vi "Main On Compile Action VI.vi"(8 "error in (no error)":errorcluster, 11 "Device Item Ref in":T1 format="%.0x") -> (0 "error out":errorcluster)   [LabVIEW 2014, in "SLSC configuration System Explorer.lvlib"]
uses:
  SLSC configuration System Explorer.lvlib
  <vilib>/NI Veristand/Custom Device API/Custom Device Item Ref.ctl
  Shared/Type Defs/SLSC compiled.ctl
  Shared/Type Defs/Res Sim compiled.ctl
  Shared/Type Defs/RT Engine Data.ctl
  Shared/Type Defs/RT IDs.ctl
  Shared/SPI Utility/Slot #.ctl
  Shared/MCP23S17/Chip Address.ctl
  Shared/Constants.vi
  <vilib>/NI Veristand/Custom Device API/Set Item Property (Variant).vi
  <vilib>/NI Veristand/Custom Device API/Custom Device API.lvlib
  Shared/SLSC configuration Shared.lvlib
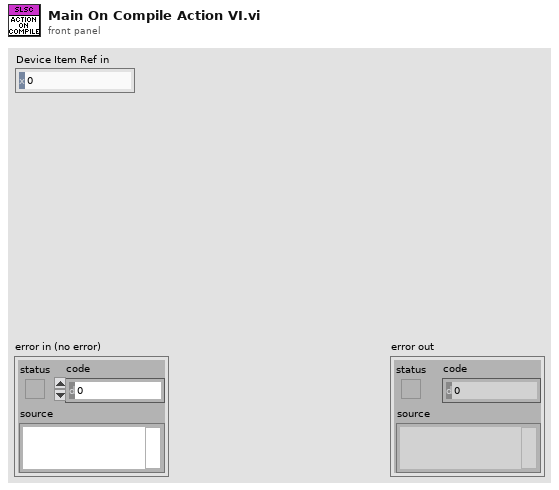
[diagram p1: front panel]
types:
  T1 = typedef "Custom Device API.lvlib/Custom Device Item Ref.ctl" = u64
  T2 = typedef "SLSC configuration Shared.lvlib/SLSC compiled.ctl" = cluster{"Initial SPI CMDs":u64[], "Res Sim data ":T3[], "Res Sim init FIFO elements":u32[], "FIU Engine Data":T4, "Battery Switch Engine Data":T4, "Wheel Speed Sensor Engine Data":T4, "Resistor Engine Data":T4, "Current Sense Engine Data":T4, "LED Engine Data":T4}
  T3 = typedef "Res Sim compiled.ctl" = cluster{"FIFO bytes3_2":u16, "Channel Old Value":dbl, "Channel data ref":i32}
  T4 = typedef "SLSC configuration Shared.lvlib/RT Engine Data.ctl" = cluster{"RT IDs":T5[], "Ordered Channels":T1[]}
  T5 = typedef "SLSC configuration Shared.lvlib/RT IDs.ctl" = cluster{"Rack #":u8, "Slot #":T6, "Chip Address (A2 A1 A0)":T7}
  T6 = typedef "SLSC configuration Shared.lvlib/Slot #.ctl" = u8
  T7 = typedef "SLSC configuration Shared.lvlib/Chip Address.ctl" = u8
  T8 = typedef "SLSC configuration Shared.lvlib/Device Settings.ctl" = cluster{"RIO Address":string, "Bitfile Path":path, "Load Delay (ms)":u32, "Divide Value":u8, "Sample Rate (S/s)":u32, "SLSC Settings":string, "SLSC FIFO Name":string}
  T9 = typedef "SLSC configuration Shared.lvlib/UEGO Compile Info.ctl" = cluster{"FPGA Item Name":string, "UEGOcalibration.<user name>":T10}
  T10 = typedef "SLSC FPGA Toolkit.lvlib/SLSC UEGO Calibration.ctl" = cluster{"Rack #":u8, "CS Bit Value/Slot #":u8, "Calibration Ticks":u32, "HW Settling Ticks":u32}
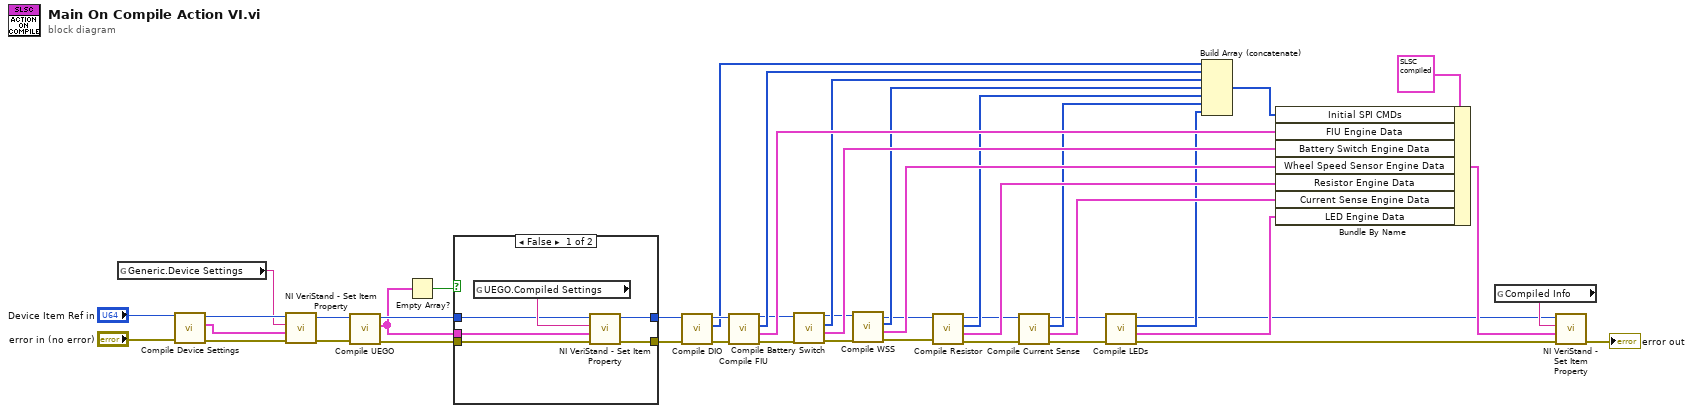
[diagram p0: block diagram]
diagram:
  n1 = global read "Constants.vi" "Generic.Device Settings"() -> (w38:string)
  n2 = call "Compile Device Settings.vi"("error in (no error)"="error in (no error)", "Device Ref in"="Device Item Ref in") -> ("error out"=w40:errorcluster, "Device Settings"=w19:T8, "Device Ref out"=w39:T1)  [unwired: 7 in]
  n3 = call-poly <vilib>:"NI VeriStand - Set Item Property.vi"("error in (no error)"=w40, "Value"=w19, "Property Name"=w38, "Item Ref in"=w39) -> ("error out"=w18:errorcluster, "Item Ref out"=w17:T1)  [unwired: 5 in, 1 out]
  n4 = call "Compile UEGO.vi"("error in (no error)"=w18, "Device Ref in"=w17) -> ("error out"=w16:errorcluster, "UEGO Calibration Info"=w12:T9[], "Device Ref out"=w13:T1)  [unwired: 7 in]
  n5 = Empty Array?(array=w12) -> (empty?=w11:bool)
  n6 = case shown="False" w11 {
    tunnel: w16 -> [w51 w53]
    tunnel: [w50 w53] -> w15
    tunnel: [w49 w54] -> w14
    tunnel: w13 -> [w48 w54]
    tunnel: w12 -> [w47 _]
    frame False {
      n7 = global read "Constants.vi" "UEGO.Compiled Settings"() -> (w52:string)
      n8 = call-poly <vilib>:"NI VeriStand - Set Item Property.vi"("error in (no error)"=w51, "Value"=w47, "Property Name"=w52, "Item Ref in"=w48) -> ("error out"=w50:errorcluster, "Item Ref out"=w49:T1)  [unwired: 5 in, 1 out]
    }
    frame True {
    }
  }
  n9 = call "Compile DIO.vi"("error in (no error)"=w15, "Device Item Ref in"=w14) -> ("error out"=w44:errorcluster, "Initial DIO SPI CMDs"=w35:u64[], "Device Item Ref out"=w43:T1)  [unwired: 7 in]
  n10 = call "Compile FIU.vi"("error in (no error)"=w44, "Device Item Ref in"=w43) -> ("error out"=w31:errorcluster, "FIU Engine Data"=w32:T4, "Initial FIU SPI CMDs"=w34:u64[], "Device Item Ref out"=w30:T1)  [unwired: 6 in]
  n11 = call "Compile Battery Switch.vi"("error in (no error)"=w31, "Device Item Ref in"=w30) -> ("error out"=w27:errorcluster, "Battery Switch Engine Data"=w28:T4, "Initial Battery Switch SPI CMDs"=w29:u64[], "Device Item Ref out"=w26:T1)  [unwired: 6 in]
  n12 = call "Compile WSS.vi"("error in (no error)"=w27, "Device Item Ref in"=w26) -> ("error out"=w23:errorcluster, "Wheel Speed Sensor Engine Data"=w24:T4, "Initial Wheel Speed Sensor SPI CMDs"=w25:u64[], "Device Item Ref out"=w22:T1)  [unwired: 6 in]
  n13 = call "Compile Resistor.vi"("error in (no error)"=w23, "Device Item Ref in"=w22) -> ("error out"=w10:errorcluster, "Resistor Engine Data"=w20:T4, "Initial Resistor SPI CMDs"=w21:u64[], "Device Item Ref out"=w9:T1)  [unwired: 6 in]
  n14 = call "Compile Current Sense.vi"("error in (no error)"=w10, "Device Item Ref in"=w9) -> ("error out"=w5:errorcluster, "Wheel Speed Sensor Engine Data"=w7:T4, "Initial Wheel Speed Sensor SPI CMDs"=w8:u64[], "Device Item Ref out"=w6:T1)  [unwired: 6 in]
  n15 = call "Compile LEDs.vi"("error in (no error)"=w5, "Device Item Ref in"=w6) -> ("error out"=w2:errorcluster, "LEDs Engine Data"=w3:T4, "Initial LEDs SPI CMDs"=w4:u64[], "Device Item Ref out"=w1:T1)  [unwired: 6 in]
  n16 = Build Array (concatenate)(w35, w34, w29, w25, w21, w8, w4) -> (w33:u64[])
  n17 = Bundle By Name(cluster=T2 {"Initial SPI CMDs"=[], "Res Sim data "=[], "Res Sim init FIFO elements"=[], "FIU Engine Data"={"RT IDs"=[], "Ordered Channels"=[]}, "Battery Switch Engine Data"={"RT IDs"=[], "Ordered Channels"=[]}, "Wheel Speed Sensor Engine Data"={"RT IDs"=[], "Ordered Channels"=[]}, "Resistor Engine Data"={"RT IDs"=[], "Ordered Channels"=[]}, "Current Sense Engine Data"={"RT IDs"=[], "Ordered Channels"=[]}, "LED Engine Data"={"RT IDs"=[], "Ordered Channels"=[]}} ("SLSC Compiled out"), "Initial SPI CMDs"=w33, "FIU Engine Data"=w32, "Battery Switch Engine Data"=w28, "Wheel Speed Sensor Engine Data"=w24, "Resistor Engine Data"=w20, "Current Sense Engine Data"=w7, "LED Engine Data"=w3) -> (w36:T2)
  n18 = global read "Constants.vi" "Compiled Info"() -> (w46:string)
  n19 = call-poly <vilib>:"NI VeriStand - Set Item Property.vi"("error in (no error)"=w2, "Value"=w36, "Property Name"=w46, "Item Ref in"=w1) -> ("error out"=→"error out":errorcluster)  [unwired: 5 in, 2 out]
